vi "Binary 저장.vi"() -> ()   [LabVIEW 2014]
uses:
  <vilib>/Analysis/1siggen.llb/General Aperiodic Triangle.vi
  <vilib>/Analysis/NI_AALBase.lvlib
panel:
  out "에러 출력":errorcluster
  out "웨이브폼 그래프":dbl[][](graph)
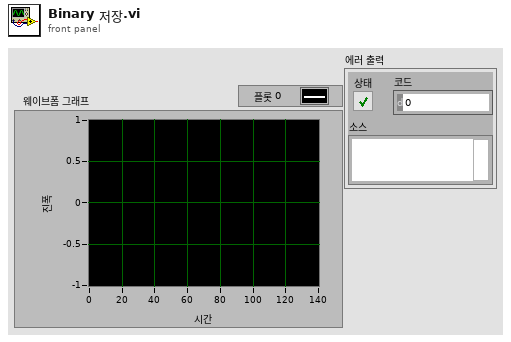
[diagram p1: front panel]
types:
  T1 = enum16{"big-endian, network order", "native, host order", "little-endian"}
  T2 = enum16{"open", "replace", "create", "open or create", "replace or create", "replace or create with confirmation"}
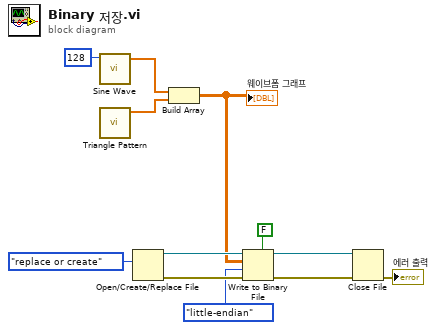
[diagram p0: block diagram]
diagram:
  n1 = call <vilib>:"Sine Wave.vi"("samples"=128) -> ("sine wave"=w12:dbl[])  [unwired: 4 in, 2 out]
  n2 = call <vilib>:"Triangle Pattern.vi"() -> ("Triangle Pattern"=w11:dbl[])  [unwired: 10 in, 1 out]
  n3 = Open/Create/Replace File(operation (0:open)=T2."replace or create" ("동작(0:open)")) -> (refnum out=w10:refnum<file>, error out=w8:errorcluster)  [unwired: 5 in, 1 out]
  n4 = Build Array(w12, w11) -> (w6:dbl[][])
  "웨이브폼 그래프" <- w6
  n5 = Write to Binary File(file (use dialog)=w10, data=w6, error in=w8, 5:FALSE ("배열 또는 문자열 크기를 앞에 추가? (참)"), 9:T1."little-endian" ("바이트 순서(0:big-endian, network order)")) -> (refnum out=w9:refnum<file>, error out=w7:errorcluster)  [unwired: 1 in, 1 out]
  n6 = Close File(refnum=w9, error in=w7) -> (error out=→"에러 출력":errorcluster)  [unwired: 1 out]
